vi "Collect Statistics.vi"(0 "VISA resource name":refnum<visa-resource-name>, 11 "error in (no error)":errorcluster) -> (4 "VISA resource name out":refnum<visa-resource-name>, 6 "standard dev":dbl format="%.2e", 8 "mean":dbl format="%.2e", 10 "peak to peak dev":dbl format="%.2e", 15 "error out":errorcluster)   [LabVIEW 2018, in "Agilent 87XX Series.lvlib"]
doc: "This VI for the HP8753B Network Analyzer reads the mean, standard deviation, and peak to peak deviation."
uses:
  Agilent 87XX Series.lvlib
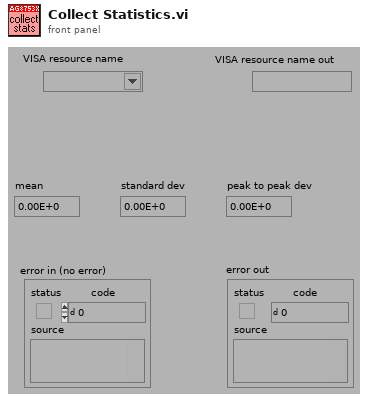
[diagram p1: front panel]
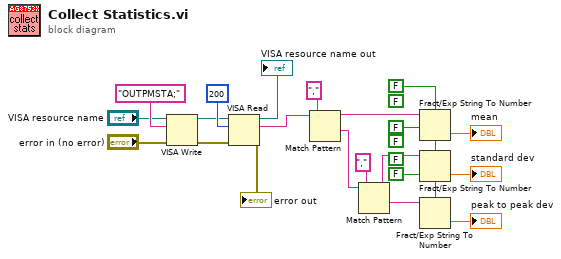
[diagram p0: block diagram]
diagram:
  (unwired) FALSE ("use system decimal point (T)")
  (unwired) FALSE ("use system decimal point (T)")
  (unwired) FALSE ("use system decimal point (T)")
  n1 = VISA Write(VISA resource name="VISA resource name", write buffer="OUTPMSTA;", error in (no error)="error in (no error)") -> (VISA resource name out=w4:refnum<visa-resource-name>, error out=w11:errorcluster)  [unwired: 1 out]
  n2 = VISA Read(VISA resource name=w4, byte count=u32 200, error in (no error)=w11) -> (VISA resource name out=→"VISA resource name out":refnum<visa-resource-name>, read buffer=w10:string, error out=→"error out":errorcluster)  [unwired: 1 out]
  n3 = Match Pattern(string=w10, regular expression=",") -> (before substring=w18:string, after substring=w19:string)  [unwired: 1 in, 2 out]
  n4 = Match Pattern(string=w19, regular expression=",") -> (before substring=w17:string, after substring=w16:string)  [unwired: 1 in, 2 out]
  n5 = Fract/Exp String To Number(use system decimal point (T)=FALSE, string=w18) -> (number=→"mean":dbl)  [unwired: 2 in, 1 out]
  n6 = Fract/Exp String To Number(use system decimal point (T)=FALSE, string=w17) -> (number=→"standard dev":dbl)  [unwired: 2 in, 1 out]
  n7 = Fract/Exp String To Number(use system decimal point (T)=FALSE, string=w16) -> (number=→"peak to peak dev":dbl)  [unwired: 2 in, 1 out]
